vi "2D Inverse Complex FFT.vi"(10 "shift?":bool, 11 "FFT {x}":cdb[][](array[numeric])) -> (0 "error":i32, 3 "X":cdb[][](array[numeric]))   [LabVIEW 2010, in "NI_AALPro.lvlib"]
doc: "Computes the inverse discrete Fourier transform (IDFT) of the input sequence <B>FFT {X}</B>. You must manually select the polymorphic instance you want to use."
uses:
  NI_AALPro.lvlib
  lvanlys.dll
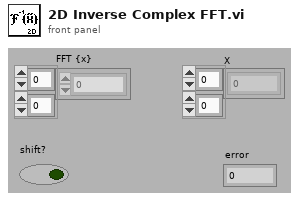
[diagram p1: front panel]
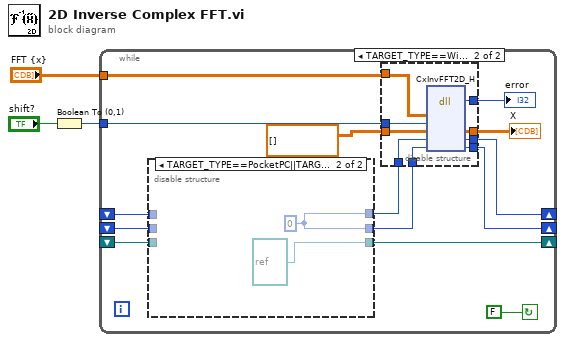
[diagram p0: block diagram]
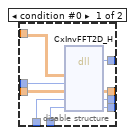
[diagram p2: hidden frame]
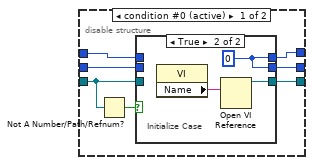
[diagram p3: hidden frame]
diagram:
  n1 = Boolean To (0,1)(Boolean="shift?") -> (0, 1=w1:i16)
  n2 = while {
    shift-left: _ -> [w15]
    shift-right: [w9] -> _
    tunnel: "FFT {x}" -> [w16]
    shift-right: [w14] -> _
    shift-left: _ -> [w13]
    shift-right: [w8] -> _
    shift-left: _ -> [w12]
    tunnel: w1 -> [w6]
    stop <- FALSE continue-if-true
    n3 = disable-structure shown="TARGET_TYPE==PocketPC||TARGET_TYPE==PalmOS||TARGET_TYPE==FPGA||TARGET_TYPE==Embedded" {
      disable-tunnel: w13 -> [w40 _]
      disable-tunnel: [w41 refnum<vi> refnum ("VI Refnum")] -> w14
      disable-tunnel: w15 -> [w39 _]
      disable-tunnel: [w38 w50] -> w10
      disable-tunnel: [w37 w50] -> w7
      disable-tunnel: w12 -> [w36 _]
      frame condition #0 (active) {
        n4 = Not A Number/Path/Refnum?(number/path/refnum=w40) -> (NaN/Path/Refnum?=w42:bool)
        n5 = case shown="True" w42 {
          tunnel: [w45 w47] -> w41
          tunnel: w40 -> [w45 _]
          tunnel: w39 -> [w44 _]
          tunnel: [w44 w48] -> w38
          tunnel: [w43 w48] -> w37
          tunnel: w36 -> [w43 _]
          frame False {
          }
          frame True {
            w48 = 0 ("error")
            # "Initialize Case"
            n6 = property class="VI"() -> ("Name"=w46:string)  [unwired: 2 in, 2 out]
            n7 = Open VI Reference(vi path=w46) -> (vi reference=w47:refnum<vi>)  [unwired: 5 in, 1 out]
          }
        }
      }
      frame condition #1 {
        w50 = 0 ("t")
      }
    }
    n8 = disable-structure shown="TARGET_TYPE==Windows||TARGET_TYPE==Mac||TARGET_TYPE==Unix" {
      disable-tunnel: w16 -> [w26 w35]
      disable-tunnel: [w25 w34] -> w11
      disable-tunnel: w10 -> [w24 w33]
      disable-tunnel: [w23 w32] -> w9
      disable-tunnel: [w22 w31] -> w8
      disable-tunnel: w7 -> [w21 w30]
      disable-tunnel: [w20 w29] -> w5
      disable-tunnel: w6 -> [w19 w28]
      disable-tunnel: cdb[][] [] ("X") -> [w18 w27]
      frame condition #0 {
        n9 = dll-call lib="C:/Program Files/National Instruments/LabVIEW 2010/resource/lvanlys.dll" fn="CxInvFFT2D_H"("FFT {x}"=w26, "shifted"=w19, w18, "tblRow"=w24, "tblCol"=w21) -> (w25:i32, w20:cdb[][], "tblRow"=w23:i32, "tblCol"=w22:i32)  [unwired: 5 in, 2 out]
      }
      frame condition #1 (active) {
        n10 = dll-call lib="C:/Program Files/National Instruments/LabVIEW 2010/resource/lvanlys.dll" fn="CxInvFFT2D_H"("xH"=w35, "shifted"=w28, "yH"=w27, "tblRow"=w33, "tblCol"=w30) -> ("return type"=w34:i32, "yH"=w29:cdb[][], "tblRow"=w32:i64, "tblCol"=w31:i64)  [unwired: 5 in, 2 out]
      }
    }
    "X" <- w5
    "error" <- w11
  }
